vi "Puma_Ground_Control_Station_V2.1.vi"(0 "?":refnum<visa-resource-name>="COM3", 1 "?":u32=9600, 9 "XON":u8=17 format="%.0x", 14 "XOFF":u8=19 format="%.0x", 15 "?":u32=10000, 21 "?":bool=TRUE, 24 "?":u8=10 format="%.0x", 25 "bsize":u32=4096) -> ()   [LabVIEW 2015]
doc: "The Advanced Serial Read and Write example performs a Serial Port Read, a Serial Port Write, or a combination of these actions while setting some advanced serial features like buffer size, termination characters, and XON/XOFF flow control. The user selects the actions (read or write) on the front panel. If both are selected, the VI will write the data first, read the data and then close the VISA session that is opened to the port. \n\nThe parameters set for the serial port must match the parameters of the connected instrument or device. In this example, the bytes to read parameter specifies the number of bytes that the serial port reads. If there were more bytes at the port than the number specified in bytes to read, those bytes would not be read. Also, if you specify to read more bytes than the number of bytes actually read, you might receive a timeout error message.\n\nINSTRUCTIONS:\n1) Select the serial resource and configuration parameters (baud rate, data bits, parity, stop bits, flow control).\n2) Termination character can be enabled and set. Also, set the required input buffer size prior to running the example.\n3) Select the operations to be performed. \n4) Connect the serial port to your device. If no device is available, perform a loopback test by doing one of the following. Short pins 2 and 3 on a RS-232 cable or short pin 4 to pin 8 and pin 5 to pin 9 on a RS-485/422 cable. \n5) Run the VI to see the data read. (The \"read string\" will match the \"string to write\" if a loopback test was performed.)\n\nThis example exposes several advanced features that you may need for your application. Not all applications need all the features shown in this example. The input buffer size is likely an important setting that you want to control in your application. This example expands upon the flow control option for XON and XOFF, allowing the user to choose those control characters. The timeout parameter has been brought to the front panel so a user can specify the time period the VISA Read will wait for the number of bytes to read before timing out. Also, the user has several controls for the termination character, which is discussed later.\n\nNote that you can press the write and read buttons and change the bytes to read parameters on the fly, while the example is running. However, you must stop the example to change the other configuration parameters after the example has started running, and then run again.\n\nSet the I/O buffer size slightly higher the amount of data you expect to receive. This is very important for applications that don't use flow control, as you may lose characters if the receive buffer overflows.\n\nSetting the timeout period ensures that the operation returns with a timeout error if the operation cannot be performed in the specified time period. \n\nSome devices require a termination character in order to identify the end of command strings. Some devices send a termination character to signify the end of data to be read. \n\nThis example shows how you can end the Read operation once a termination character is detected in the buffer and/or append a termination character at the end of the Write data. To enable the Read to end on a termination character, use the VISA Configure Serial Port or use the VISA Properties Serial End Mode for Reads, Termination Character Enable, and Termination Character. To end the Write with a termination character, use the VISA Properties Serial End Mode for Writes, the Send End Enable, and Termination Character. In this example, the same termination character is used for both the Read and the Write. You can specify two different characters for your application, if desired.\n\nYour application may require specific characters for the XON/XOFF Flow Control. You can specify these characters with the VISA Properties Flow Control XOFF Character and Flow Control XON Character. Note that if the standard XON and XOFF characters are used, then decimal 17 and 19 are unavailable for data values. Remember that using flow control and setting an adequate buffer size allow you to prevent buffer overflows."
uses:
  <vilib>/Instr/_visa.llb/VISA Configure Serial Port (Instr).vi
panel:
  in  "Fan Shutdown":bool
  in  "DValve / AV6-T":bool
  in  "Flight Control Board":bool
  in  "Safety":bool
  in  "Test Run":bool
  in  "Reset Control":bool
  in  "Primary Safety 2":bool
  out "?":bool
  out "Motors":cluster{dbl, dbl, dbl, dbl}(graph)={1000.0, 1000.0, 1000.0, 1000.0}
  in  "Pressure Transducers":T1(tab)
  out "?":cluster{dbl, dbl, dbl, dbl, dbl}(graph)
  out "?":cluster{dbl, dbl}(graph)
  in  "Thermocouples":T2(tab)
  out "?":cluster{dbl, dbl, dbl, dbl}(graph)
  out "?":cluster{dbl, dbl}(graph)
  out "fo-u":bool
  out "av5-m":bool
  out "fc-u":bool
  out "PT1-U > 5000 PSI":bool
  out "Takeoff Started":bool
  out "Iterations":i32
  out "Reset Triggered":bool
  in  "PixHawk":bool
  in  "XON 2":u8=17 format="%.0x"
  in  "XOFF 2":u8=19 format="%.0x"
  in  "?":bool=TRUE
  in  "bsize 2":u32=4096
  in  "?":u8=10 format="%.0x"
  in  "?":bool=TRUE
  in  "?":u32=10000
  in  "?":refnum<visa-resource-name>="COM3"
  in  "?":u32=9600
  out "Max Values":T3={20.764332288, 0.0, 0.0, 0.0, 0.0, 0.0, 0.0, 201.058, 25.138999999999953, 0.0, 57.16000000000008, 0.0, 8.920000000000016, 15.403999999999996}
  in  "Data Filename":string
  out "Offset 7":dbl=-251.3
  out "Multiplier 7":dbl=1.264
  out "Offset 6":dbl=-250.2
  out "Offset 5":dbl=-250.3
  out "Offset 4":dbl=-1253.0
  out "Offset 3":dbl=-250.9
  out "Offset 2":dbl=-249.8
  out "Offset 1":dbl=-251.0
  out "Multiplier 6":dbl=1.264
  out "Multiplier 5":dbl=1.277
  out "Multiplier 4":dbl=6.36
  out "Multiplier 3":dbl=1.274
  out "Multiplier 2":dbl=1.267
  out "Multiplier 1":dbl=1.277
  in  "Begin Checklist":bool
  out "Manual Abort Tested":bool
  out "Flight Control On":bool
  out "Reset Triggered 2":bool
  out "Primary Safety Active":bool
  out "Craft Triggered Softkill Active":bool
  out "Hardkill Active":bool
  out "ms":dbl=163640.0
  out "vcc 6":bool
  out "gnd 6":bool=TRUE
  out "TC6":bool
  out "vcc 5":bool
  out "gnd 5":bool=TRUE
  out "TC5":bool
  out "vcc 4":bool
  out "gnd 4":bool=TRUE
  out "TC4":bool
  out "vcc 3":bool
  out "gnd 3":bool=TRUE
  out "TC3":bool
  out "vcc 2":bool
  out "gnd 2":bool=TRUE
  out "TC2":bool
  out "vcc":bool
  out "gnd":bool=TRUE
  out "TC1":bool
  out "Engine 4":dbl=1000.0
  out "Engine 3":dbl=1000.0
  out "Engine 2":dbl=1000.0
  out "Engine 1":dbl=1000.0
  out "soft kill ind":bool
  out "dump fuel ind":bool
  out "abort ind":bool
  out "run ind":bool
  out "av6-t ind":bool
  out "Control input":bool
  out "return":bool
  out "Control (on/off)":bool
  out "PT5-M":dbl=-6.084000000000003
  out "PT2-M":dbl=-10.039999999999992
  out "PT2-U":dbl=-250.3
  out "PT1-U":dbl=-38.24000000000001
  out "PT3-M":dbl=-141.336
  out "PT1-M":dbl=9.934999999999945
  out "PT4-M":dbl=181.90299999999996
  out "TCp-2":dbl=-2.0
  out "TCp-1":dbl=-2.0
  out "TCpw-4":dbl=-2.0
  out "TCpw-3":dbl=-2.0
  out "TCpw-2":dbl=-2.0
  out "TCpw-1":dbl=-2.0
  out "Output":string="h:;"
  in  "?":enum32{"Test"}(tab)
  in  "Primary Safety":bool=TRUE
  in  "Soft Kill":bool
  in  "Simulate":bool
  in  "Reset FC":bool
  in  "Full Power":bool
  in  "Secondary Safety":bool=TRUE
  in  "Takeoff":bool
  in  "Calibrate":bool
  in  "abort":bool
  out "?":dbl(graph)=20.40794784
  in  "Send":bool=TRUE
  in  "Recieve":bool=TRUE
  in  "bytes to read 2":u32=1000
  out "?":u32=107
  out "?":string[](array[string])=["339", "205", "86", "191", "0", "190", "194", "-2.00", "-2.00", "-2.00", "-2.00", "-2.00", "-2.00", "555", "1000", "1000", "1000", "1000", "163640"]
  out "?":string[](array[string])=["p:339,205,86,191,0,190,194", "t:-2.00,-2.00,-2.00,-2.00,-2.00,-2.00", "v:555", "m:1000,1000,1000,1000", "h:", "s:163640", ""]
  out "Voltage Sensor":dbl=20.40794784
  in  "dump fuel":bool
  in  "?":enum32{"Ignore"}(tab)
  out "?":bool=TRUE
  out "String":string
  in  "String 3":string
  in  "?":bool=TRUE
  in  "tank iso":bool
  in  "Av-6Tt":bool
  in  "FC-U Toggle":bool
  in  "FOU":bool
  out "?":dbl(slide) scale=0.2..200.0
  out "FO-U":bool
  out "FC-U":bool
  out "AV6-T":bool
  out "AV1-T":bool
  out "AV3-T":bool
  out "AV4-T":bool
  out "AV5-T":bool
  out "AV2-T":bool
  # "Data From Craft:"
  # "FO-U"
  # "FC-U"
  # "receive"
  # "send"
  # "AV6-M"
  # "AV5-M"
  # "green=open - check thermocouple attachments\nred=short gnd - contact Power or GNC\nblue=short vcc - contact Power or GNC"
  # "AV1-M"
  # "AV2-M"
  # "AV3-M"
  # "AV4-M"
  # "Voltage"
  # "TCp2-M"
  # "Tcw1-E"
  # "TCp1-M"
  # "TCw4-E"
  # "TCw3-E"
  # "TCw2-E"
  # "PT4-M"
  # "PT1-M"
  # "PT3-M"
  # "PT1-U"
  # "PT2-U"
  # "PT2-M"
  # "PT5-M"
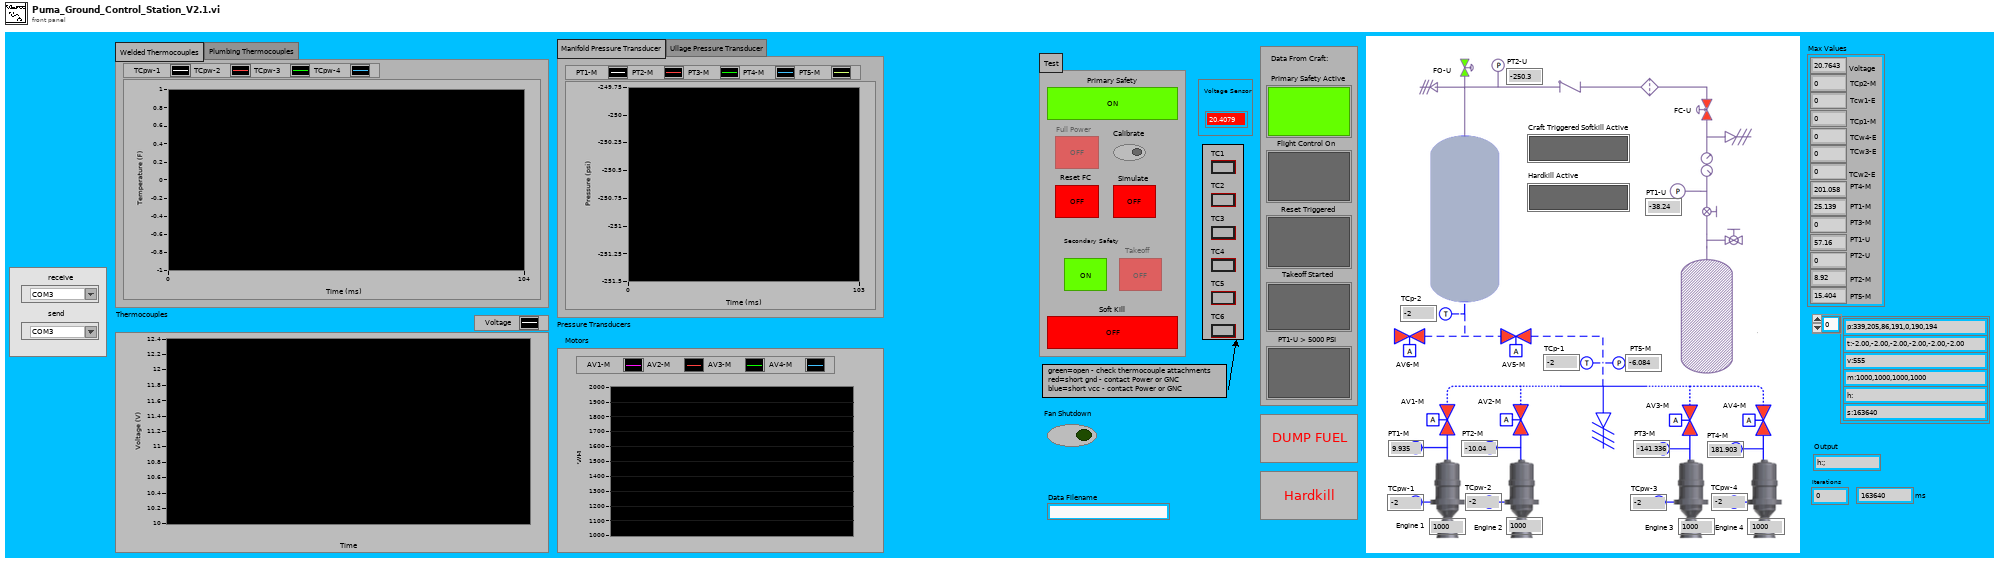
[diagram p1: front panel]
types:
  T1 = enum32{"Manifold Pressure Transducer", "Ullage Pressure Transducer"}
  T2 = enum32{"Welded Thermocouples", "Plumbing Thermocouples"}
  T3 = cluster{dbl, dbl, dbl, dbl, dbl, dbl, dbl, dbl, dbl, dbl, dbl, dbl, dbl, dbl}
  T4 = enum16{"open", "replace", "create", "open or create", "replace or create", "replace or create with confirmation"}
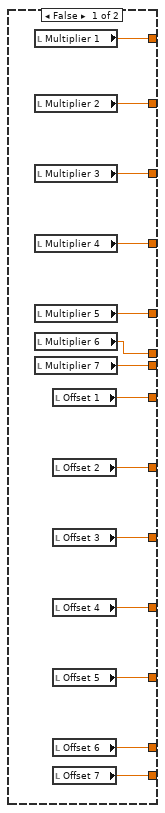
[diagram p3: hidden frame]
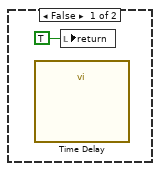
[diagram p13: hidden frame]
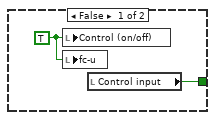
[diagram p16: hidden frame]
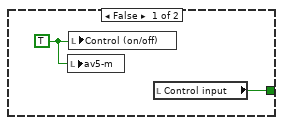
[diagram p18: hidden frame]
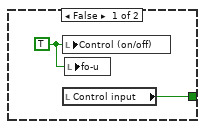
[diagram p20: hidden frame]
diagram:
  w2 = TRUE
  w1 = FALSE
  w51 = u16 16  # I/O Receive Buffer mask
  w75 = u16 16  # I/O Receive Buffer mask
  # "Comment"
  # "Set default values"
  n1 = while {
    stop <- FALSE stop-if-true
    n2 = case shown="True" "Calibrate" {
      tunnel: [w109 w123] -> w93
      tunnel: [w108 w122] -> w92
      tunnel: [w107 w121] -> w91
      tunnel: [w106 w120] -> w90
      tunnel: [w105 w119] -> w89
      tunnel: [w104 w118] -> w88
      tunnel: [w103 w117] -> w87
      tunnel: [w101 w116] -> w86
      tunnel: [w102 w115] -> w85
      tunnel: [w100 w114] -> w84
      tunnel: [w99 w113] -> w83
      tunnel: [w98 w112] -> w82
      tunnel: [w97 w111] -> w81
      tunnel: [w96 w110] -> w80
      frame False {
        n3 = local read "Multiplier 1"() -> (w109:dbl)
        n4 = local read "Multiplier 2"() -> (w108:dbl)
        n5 = local read "Multiplier 3"() -> (w107:dbl)
        n6 = local read "Multiplier 4"() -> (w106:dbl)
        n7 = local read "Multiplier 5"() -> (w105:dbl)
        n8 = local read "Multiplier 6"() -> (w104:dbl)
        n9 = local read "Multiplier 7"() -> (w103:dbl)
        n10 = local read "Offset 1"() -> (w101:dbl)
        n11 = local read "Offset 2"() -> (w102:dbl)
        n12 = local read "Offset 3"() -> (w100:dbl)
        n13 = local read "Offset 4"() -> (w99:dbl)
        n14 = local read "Offset 5"() -> (w98:dbl)
        n15 = local read "Offset 6"() -> (w97:dbl)
        n16 = local read "Offset 7"() -> (w96:dbl)
      }
      frame True {
        n17 = call "P configure.vi"() -> ("Multiplier 1"=w123:dbl, "Offset 1"=w116:dbl, "Multiplier 2"=w122:dbl, "Offset 2"=w115:dbl, "Multiplier 3"=w121:dbl, "Offset 6"=w111:dbl, "Offset 3"=w114:dbl, "Offset 7"=w110:dbl, "Multiplier 4"=w120:dbl, "Multiplier 7"=w117:dbl, "Multiplier 6"=w118:dbl, "Offset 5"=w112:dbl, "Multiplier 5"=w119:dbl, "Offset 4"=w113:dbl)  [unwired: 2 in]
      }
    }
    "Multiplier 1" <- w93
    "Multiplier 2" <- w92
    "Multiplier 3" <- w91
    "Multiplier 4" <- w90
    "Multiplier 5" <- w89
    "Offset 1" <- w86
    "Offset 2" <- w85
    "Offset 3" <- w84
    "Offset 4" <- w83
    "Offset 5" <- w82
    "Offset 6" <- w81
    "Multiplier 7" <- w87
    "Offset 7" <- w80
    "Multiplier 6" <- w88
  }
  n18 = while {
    stop <- FALSE stop-if-true
    n19 = local read "Control (on/off)"() -> (w126:bool)
    n20 = Wait Until Next ms Multiple(millisecond multiple=50) -> ()  [unwired: 1 out]
    n21 = case shown="True" w126 {
      frame False {
      }
      frame True {
        n22 = local read "dump fuel ind"() -> (w142:bool)
        n23 = local read "soft kill ind"() -> (w140:bool)
        n24 = local read "av6-t ind"() -> (w143:bool)
        n25 = local read "abort ind"() -> (w144:bool)
        n26 = local read "fc-u"() -> (w130:bool)
        n27 = local read "av5-m"() -> (w132:bool)
        n28 = local read "fo-u"() -> (w134:bool)
        n29 = local read "run ind"() -> (w141:bool)
        n30 = case shown="True" w140 {
          tunnel: [_ "Are you sure you want to Softkill?"] -> w135
          frame False {
          }
          frame True {
          }
        }
        n31 = case shown="True" w142 {
          tunnel: [_ "Are you sure you want to Dump Fuel?"] -> w137
          frame False {
          }
          frame True {
          }
        }
        n32 = case shown="True" w143 {
          tunnel: [_ "Are you sure you want to Open AV6-M?"] -> w138
          frame False {
          }
          frame True {
          }
        }
        n33 = case shown="True" w144 {
          tunnel: [_ "Are you sure you want to Abort?"] -> w139
          frame False {
          }
          frame True {
          }
        }
        n34 = case shown="True" w134 {
          tunnel: [_ "Are you sure you want to open FO-U?"] -> w133
          frame False {
          }
          frame True {
          }
        }
        n35 = case shown="True" w130 {
          tunnel: [_ "Are you sure you want to open FC-U?"] -> w129
          frame False {
          }
          frame True {
          }
        }
        n36 = case shown="True" w132 {
          tunnel: [_ "Are you sure you want to open AV5-M?"] -> w131
          frame False {
          }
          frame True {
          }
        }
        n37 = case shown="True" w141 {
          tunnel: [_ "Are you sure you want to Run?"] -> w136
          frame False {
          }
          frame True {
          }
        }
        n38 = Concatenate Strings(w135, w136, w137, w138, w139, w133, w131, w129) -> (w128:string)
        n39 = call "DialogBoxSubVI.vi"("Prompt"=w128) -> ("Boolean"=w127:bool)  [unwired: 9 in]
        n40 = case shown="True" w127 {
          frame False {
            n41 = call "Time Delay"() -> ()  [unwired: 11 in, 1 out]
            n42 = local write "return"(TRUE) -> ()
          }
          frame True {
            n43 = call "Time Delay2"() -> ()  [unwired: 11 in, 1 out]
            n44 = local write "return"(TRUE) -> ()
          }
        }
        n45 = local write "Control input"(w127) -> ()
      }
    }
  }
  n46 = call-poly "VISA Configure Serial Port"("VISA resource name"="?", "timeout (10sec)"="?", "termination char\n(0xA = '\\n' = LF)"="?", "Enable Termination\nChar (T)"="?", "baud rate (9600)"="?") -> ("VISA resource name out"=w64:refnum<visa-resource-name>, "error out"=w67:errorcluster)  [unwired: 5 in, 4 out]
  n47 = call-poly "VISA Configure Serial Port"("VISA resource name"="?", "timeout (10sec)"="?", "termination char\n(0xA = '\\n' = LF)"="?", "Enable Termination\nChar (T)"="?", "baud rate (9600)"="?") -> ("VISA resource name out"=w40:refnum<visa-resource-name>, "error out"=w43:errorcluster)  [unwired: 5 in, 4 out]
  n48 = case shown="True" "?" {
    selector: "?" -> [_ w157]
    tunnel: w64 -> [w155 w163]
    tunnel: w67 -> [w156 w162]
    tunnel: [w155 w161] -> w65
    tunnel: [w156 w160] -> w66
    tunnel: "?" -> [_ w158]
    frame False {
    }
    frame True {
      w159 = u16 2 items=["None", "LastBit", "TermChar", "Break"] ("Serial Settings:Serial End Mode for Writes")
      n49 = property class="Instr"(reference=w163, error in=w162, "Serial Settings:End Mode for Writes"=w159, "Message Based Settings:Send End Enable"=w157, "Message Based Settings:Termination Character"=w158) -> (reference out=w161:refnum<visa-resource-name>, error out=w160:errorcluster)
    }
  }
  n50 = case shown="True" "?" {
    selector: "?" -> [_ w166]
    tunnel: w40 -> [w164 w172]
    tunnel: w43 -> [w165 w171]
    tunnel: [w164 w170] -> w41
    tunnel: [w165 w169] -> w42
    tunnel: "?" -> [_ w167]
    frame False {
    }
    frame True {
      w168 = u16 2 items=["None", "LastBit", "TermChar", "Break"] ("Serial Settings:Serial End Mode for Writes")
      n51 = property class="Instr"(reference=w172, error in=w171, "Serial Settings:End Mode for Writes"=w168, "Message Based Settings:Send End Enable"=w166, "Message Based Settings:Termination Character"=w167) -> (reference out=w170:refnum<visa-resource-name>, error out=w169:errorcluster)
    }
  }
  n52 = property on="Secondary Safety" class="Bool (strict)"("Value"=w2) -> ()  [unwired: 2 in, 2 out]
  n53 = property on="Primary Safety" class="Bool (strict)"("Value"=w2) -> ()  [unwired: 2 in, 2 out]
  n54 = property on="Reset FC" class="Bool (strict)"("Value"=w1) -> ()  [unwired: 2 in, 2 out]
  n55 = property on="Simulate" class="Bool (strict)"("Value"=w1) -> ()  [unwired: 2 in, 2 out]
  n56 = property on="Craft Triggered Softkill Active" class="Bool (strict)"("Value"=w1) -> ()  [unwired: 2 in, 2 out]
  n57 = property on="Hardkill Active" class="Bool (strict)"("Value"=w1) -> ()  [unwired: 2 in, 2 out]
  n58 = property on="Takeoff Started" class="Bool (strict)"("Value"=w1) -> ()  [unwired: 2 in, 2 out]
  n59 = property on="FOU" class="Bool (strict)"("Value"=w1) -> ()  [unwired: 2 in, 2 out]
  n60 = property on="Soft Kill" class="Bool (strict)"("Value"=w1) -> ()  [unwired: 2 in, 2 out]
  n61 = property on="dump fuel" class="Bool (strict)"("Value"=w1) -> ()  [unwired: 2 in, 2 out]
  n62 = property on="abort" class="Bool (strict)"("Value"=w1) -> ()  [unwired: 2 in, 2 out]
  n63 = property on="Manual Abort Tested" class="Bool (strict)"("Value"=w1) -> ()  [unwired: 2 in, 2 out]
  n64 = Build Path(base path=path "C:/Users/Lunar Lion/Desktop/Puma_Test_Data" ("file path (use dialog)"), name or relative path="Data Filename") -> (appended path=w59:path)
  n65 = Build Array("PT4-M_a", "PT1-M_a", "PT3-M_a", "PT1-U_a", "PT2-U_a", "PT2-M_a", "PT5-M_a", "PT4-M", "PT1-M", "PT3-M", "PT1-U", "PT2-U", "PT2-M", "PT5-M", "TCp2-M", "TCw1-E", "TCp1-M", "TCw4-E", "TCw3-E", "TCw2-E", "Voltage", "Motor1", "Motor2", "Motor3", "Motor4", "Statestring") -> (w12:string[])
  n66 = VISA Set I/O Buffer Size(VISA resource name=w65, mask (16)=w75, size (4096)="bsize", error in (no error)=w66) -> (VISA resource name out=w71:refnum<visa-resource-name>, error out=w70:errorcluster)
  n67 = VISA Set I/O Buffer Size(VISA resource name=w41, mask (16)=w51, size (4096)="bsize 2", error in (no error)=w42) -> (VISA resource name out=w47:refnum<visa-resource-name>, error out=w46:errorcluster)
  n68 = Open/Create/Replace File(file path (use dialog)=w59, operation (0:open)=T4."replace or create with confirmation") -> (refnum out=w9:refnum<file>)  [unwired: 4 in, 2 out]
  n69 = Array To Spreadsheet String(array=w12, 3:"%s" ("format string")) -> (spreadsheet string=w10:string)  [unwired: 1 in]
  n70 = property class="Instr"(reference=w71, error in=w70, "Serial Settings:Flow Control XON Character"="XON", "Serial Settings:Flow Control XOFF Character"="XOFF") -> (reference out=w63:refnum<visa-resource-name>, error out=w62:errorcluster)
  n71 = property class="Instr"(reference=w47, error in=w46, "Serial Settings:Flow Control XON Character"="XON 2", "Serial Settings:Flow Control XOFF Character"="XOFF 2") -> (reference out=w39:refnum<visa-resource-name>)  [unwired: 1 out]
  n72 = Write to Text File(file (use dialog)=w9, text=w10) -> (refnum out=w8:refnum<file>)  [unwired: 2 in, 2 out]
  n73 = while {
    tunnel: w63 -> [w304]
    tunnel: w62 -> [w373]
    tunnel: [w283] -> w7
    tunnel: [w282] -> w61
    shift-right: [w473] -> _
    shift-left: _ -> [w472]
    shift-right: [w184] -> _
    shift-left: _ -> [w434]
    shift-right: [w442] -> _
    shift-left: _ -> [w443]
    shift-right: [w433] -> _
    shift-left: _ -> [w457]
    shift-right: [w187] -> _
    shift-left: _ -> [w455]
    shift-right: [w435] -> _
    shift-left: _ -> [w438]
    shift-right: ["Begin Checklist"] -> _
    shift-left: _ -> [w354]
    tunnel: w8 -> [w326]
    tunnel: [w323] -> w58
    shift-right: [w307] -> _
    shift-left: T3 {0.0, 0.0, 0.0, 0.0, 0.0, 0.0, 0.0, 0.0, 0.0, 0.0, 0.0, 0.0, 0.0, 0.0} -> [w306]
    tunnel: w39 -> [_]
    shift-right: [w182] -> _
    shift-left: _ -> [w186]
    shift-right: [w179] -> _
    shift-left: _ -> [w180]
    shift-right: [w176] -> _
    shift-left: _ -> [w177]
    i -> [w292]
    stop <- FALSE stop-if-true
    w208 = u32 13816530
    w212 = 120.0
    w218 = 1200.0
    w209 = u32 16776704
    w225 = 800.0
    # "The purpose of this indicator is not entirely clear"
    # "Hidden test run button."
    # "Hidden secondary safety."
    # "Hidden reset control button."
    # "Hidden flight control board button."
    # "Un-named indicator, hidden."
    # "Hidden dump valve indicator/button?"
    # "Hidden primary safety"
    # "Tabs for the main command buttons."
    # "Ignore tab with the two strings and indicator light."
    # "Above nominal thresholds:\n   All PTs except PT1-U: 800\n   TCpw-1 to 4: 1200\n   TCp-1 and 2: 120"
    # "The second String \nParsing Indicator"
    # "String Parsing Indicator control"
    # "ENSURE THE PTs ARE HOOKED UP PROPERLY"
    # "Here, if PT1-U indicates a pressure greater than 5000 psi,\nthe indicator represented in the case structure is turned green. Otherwise, it is turned red."
    # "FO-U Case"
    # "AV6 -T Case"
    # "AV5-T Case"
    # "AV5-T Toggle"
    n74 = case shown="True" FALSE {
      frame False {
      }
      frame True {
        w589 = FALSE
        n75 = local write "FOU"(TRUE) -> ()
        n76 = local write "AV1-T"(w589) -> ()
        n77 = local write "AV2-T"(w589) -> ()
        n78 = local write "AV3-T"(w589) -> ()
        n79 = local write "AV4-T"(w589) -> ()
        n80 = local write "FC-U Toggle"(w589) -> ()
        n81 = local write "tank iso"(w589) -> ()
      }
    }
    n82 = property on="abort" class="Bool (strict)"() -> ("Value"=w260:bool)  [unwired: 2 in, 2 out]
    n83 = property on="Voltage Sensor" class="DigNum (strict)"("NumText.TextColor"=u32 16448250) -> ()  [unwired: 2 in, 2 out]
    n84 = local read "Voltage Sensor"() -> (w264:dbl)
    n85 = case shown="False" w260 {
      frame False {
        n86 = property on="Soft Kill" class="Bool (strict)"() -> ("Value"=w573:bool)  [unwired: 2 in, 2 out]
        n87 = case shown="True" w573 {
          frame False {
            n88 = property on="dump fuel" class="Bool (strict)"("DisabledEnum"=0) -> ()  [unwired: 2 in, 2 out]
          }
          frame True {
            n89 = property on="dump fuel" class="Bool (strict)"("DisabledEnum"=2) -> ()  [unwired: 2 in, 2 out]
          }
        }
      }
      frame True {
        n90 = property on="dump fuel" class="Bool (strict)"("DisabledEnum"=2) -> ()  [unwired: 2 in, 2 out]
      }
    }
    n91 = Greater Than 0?(x=w264) -> (x > 0?=w271:bool)
    n92 = Less?(x=w264, y=14.0) -> (x < y?=w277:bool)
    n93 = Less?(x=w264, y=13.0) -> (x < y?=w272:bool)
    n94 = Greater?(x=w264, y=13.0) -> (0:w276:bool)
    n95 = Greater?(x=w264, y=14.0) -> (0:w268:bool)
    n96 = Less?(x=w264, y=15.5) -> (x < y?=w269:bool)
    n97 = Greater?(x=w264, y=15.5) -> (0:w263:bool)
    n98 = And(x=w268, y=w269) -> (x .and. y?=w267:bool)
    n99 = And(x=w271, y=w272) -> (x .and. y?=w273:bool)
    n100 = And(x=w276, y=w277) -> (x .and. y?=w278:bool)
    n101 = case shown="True" w273 {
      frame False {
      }
      frame True {
        n102 = property on="Voltage Sensor" class="DigNum (strict)"("NumText.BGColor"=u32 16714752) -> ()  [unwired: 2 in, 2 out]
      }
    }
    n103 = case shown="True" w278 {
      frame False {
      }
      frame True {
        n104 = property on="Voltage Sensor" class="DigNum (strict)"("NumText.BGColor"=u32 16757522) -> ()  [unwired: 2 in, 2 out]
        n105 = property on="Voltage Sensor" class="DigNum (strict)"("NumText.TextColor"=u32 16777222) -> ()  [unwired: 2 in, 2 out]
      }
    }
    n106 = case shown="True" w267 {
      frame False {
      }
      frame True {
        n107 = property on="Voltage Sensor" class="DigNum (strict)"("NumText.BGColor"=u32 6618880) -> ()  [unwired: 2 in, 2 out]
        n108 = property on="Voltage Sensor" class="DigNum (strict)"("NumText.TextColor"=u32 16777222) -> ()  [unwired: 2 in, 2 out]
      }
    }
    n109 = case shown="True" w263 {
      frame False {
      }
      frame True {
        n110 = property on="Voltage Sensor" class="DigNum (strict)"("NumText.BGColor"=u32 15876863) -> ()  [unwired: 2 in, 2 out]
      }
    }
    n111 = Exclusive Or(1:w457, 2:"abort") -> (0:w459:bool)
    n112 = case shown="True" w459 {
      tunnel: [w653 w655] -> w433
      tunnel: w457 -> [w653 w654]
      frame False {
      }
      frame True {
        n113 = case shown="False" w654 {
          tunnel: [w656 FALSE ("T button?")] -> w655
          frame False {
            w657 = TRUE
            n114 = local write "abort ind"(w657) -> ()
            n115 = local write "Control (on/off)"(w657) -> ()
            n116 = local read "Control input"() -> (w656:bool)
          }
          frame True {
          }
        }
      }
    }
    n117 = Exclusive Or(1:w438, 2:"Soft Kill") -> (0:w436:bool)
    n118 = Exclusive Or(1:w455, 2:"dump fuel") -> (0:w456:bool)
    n119 = case shown="True" w436 {
      tunnel: [w643 w645] -> w435
      tunnel: w438 -> [w643 w644]
      frame False {
      }
      frame True {
        n120 = case shown="False" w644 {
          tunnel: [w646 _] -> w645
          frame False {
            w647 = TRUE
            n121 = local write "soft kill ind"(w647) -> ()
            n122 = local write "Control (on/off)"(w647) -> ()
            n123 = local read "Control input"() -> (w646:bool)
          }
          frame True {
          }
        }
      }
    }
    n124 = case shown="True" w456 {
      tunnel: [w648 w650] -> w187
      tunnel: w455 -> [w648 w649]
      frame False {
      }
      frame True {
        n125 = case shown="False" w649 {
          tunnel: [w652 _] -> w650
          frame False {
            w651 = TRUE
            n126 = local write "Control (on/off)"(w651) -> ()
            n127 = local write "dump fuel ind"(w651) -> ()
            n128 = local read "Control input"() -> (w652:bool)
          }
          frame True {
          }
        }
      }
    }
    n129 = Not(x="Secondary Safety") -> (.not. x?=w293:bool)
    n130 = property on="TCpw-1" class="DigNum (strict)"() -> ("Value"=w222:dbl)  [unwired: 2 in, 2 out]
    n131 = property on="TCpw-2" class="DigNum (strict)"() -> ("Value"=w217:dbl)  [unwired: 2 in, 2 out]
    n132 = property on="TCpw-3" class="DigNum (strict)"() -> ("Value"=w216:dbl)  [unwired: 2 in, 2 out]
    n133 = property on="TCpw-4" class="DigNum (strict)"() -> ("Value"=w215:dbl)  [unwired: 2 in, 2 out]
    n134 = property on="TCp-2" class="DigNum (strict)"() -> ("Value"=w210:dbl)  [unwired: 2 in, 2 out]
    n135 = property on="TCp-1" class="DigNum (strict)"() -> ("Value"=w211:dbl)  [unwired: 2 in, 2 out]
    n136 = property on="PT2-M" class="DigNum (strict)"() -> ("Value"=w235:dbl)  [unwired: 2 in, 2 out]
    n137 = property on="PT1-M" class="DigNum (strict)"() -> ("Value"=w236:dbl)  [unwired: 2 in, 2 out]
    n138 = property on="PT3-M" class="DigNum (strict)"() -> ("Value"=w234:dbl)  [unwired: 2 in, 2 out]
    n139 = property on="PT4-M" class="DigNum (strict)"() -> ("Value"=w233:dbl)  [unwired: 2 in, 2 out]
    n140 = property on="PT5-M" class="DigNum (strict)"() -> ("Value"=w227:dbl)  [unwired: 2 in, 2 out]
    n141 = property on="PT2-U" class="DigNum (strict)"() -> ("Value"=w226:dbl)  [unwired: 2 in, 2 out]
    n142 = And(x="Safety", y="Test Run") -> (x .and. y?=w488:bool)
    n143 = And(x=w293, y="Takeoff") -> (x .and. y?=w487:bool)
    n144 = Not(x="Secondary Safety") -> (.not. x?=w295:bool)
    n145 = Greater Or Equal?(x=w210, y=w212) -> (x >= y?=w213:bool)
    n146 = Greater Or Equal?(x=w211, y=w212) -> (x >= y?=w214:bool)
    n147 = Greater Or Equal?(x=w222, y=w218) -> (x >= y?=w223:bool)
    n148 = Greater Or Equal?(x=w217, y=w218) -> (x >= y?=w221:bool)
    n149 = Greater Or Equal?(x=w216, y=w218) -> (x >= y?=w220:bool)
    n150 = Greater Or Equal?(x=w215, y=w218) -> (x >= y?=w219:bool)
    n151 = Greater Or Equal?(x=w235, y=w225) -> (x >= y?=w231:bool)
    n152 = Greater Or Equal?(x=w236, y=w225) -> (x >= y?=w232:bool)
    n153 = Greater Or Equal?(x=w234, y=w225) -> (x >= y?=w230:bool)
    n154 = Greater Or Equal?(x=w233, y=w225) -> (x >= y?=w229:bool)
    n155 = Greater Or Equal?(x=w227, y=w225) -> (x >= y?=w228:bool)
    n156 = Greater Or Equal?(x=w226, y=w225) -> (x >= y?=w224:bool)
    n157 = case shown="True" "Recieve" {
      tunnel: w373 -> [w707 w712]
      tunnel: w304 -> [w708 w711]
      tunnel: [w707 w714] -> w282
      tunnel: [w708 w713] -> w283
      tunnel: [_ w710] -> _
      tunnel: [_ w709] -> w325
      frame False {
      }
      frame True {
        n158 = case "Read bytes from port." shown="No Error" w712 {
          selector: w712 -> [w717 w723]
          tunnel: [w720 w723] -> w714
          tunnel: [w721 w722] -> w713
          tunnel: w711 -> [w718 w722]
          tunnel: [w715 _] -> w710
          tunnel: [w715 _] -> w709
          frame No Error {
            n159 = VISA Read(VISA resource name=w718, byte count="bytes to read 2", error in (no error)=w717) -> (VISA resource name out=w721:refnum<visa-resource-name>, read buffer=w715:string, return count=→"?":u32, error out=w720:errorcluster)
          }
          frame Error {
          }
        }
      }
    }
    n160 = case shown="False" w295 {
      tunnel: [2 0] -> w294
      frame False {
      }
      frame True {
      }
    }
    n161 = Or(x=w487, y=w488) -> (x .or. y?=w462:bool)
    n162 = case shown="True" w213 {
      tunnel: w209 -> [_ w550]
      tunnel: w208 -> [w549 _]
      frame False {
        n163 = property on="TCp-2" class="DigNum (strict)"("NumText.BGColor"=w549) -> ()  [unwired: 2 in, 2 out]
      }
      frame True {
        n164 = property on="TCp-2" class="DigNum (strict)"("NumText.BGColor"=w550) -> ()  [unwired: 2 in, 2 out]
      }
    }
    n165 = case shown="True" w214 {
      tunnel: w209 -> [_ w552]
      tunnel: w208 -> [w551 _]
      frame False {
        n166 = property on="TCp-1" class="DigNum (strict)"("NumText.BGColor"=w551) -> ()  [unwired: 2 in, 2 out]
      }
      frame True {
        n167 = property on="TCp-1" class="DigNum (strict)"("NumText.BGColor"=w552) -> ()  [unwired: 2 in, 2 out]
      }
    }
    n168 = case shown="True" w223 {
      tunnel: w209 -> [_ w560]
      tunnel: w208 -> [w559 _]
      frame False {
        n169 = property on="TCpw-1" class="DigNum (strict)"("NumText.BGColor"=w559) -> ()  [unwired: 2 in, 2 out]
      }
      frame True {
        n170 = property on="TCpw-1" class="DigNum (strict)"("NumText.BGColor"=w560) -> ()  [unwired: 2 in, 2 out]
      }
    }
    n171 = case shown="True" w221 {
      tunnel: w209 -> [_ w558]
      tunnel: w208 -> [w557 _]
      frame False {
        n172 = property on="TCpw-2" class="DigNum (strict)"("NumText.BGColor"=w557) -> ()  [unwired: 2 in, 2 out]
      }
      frame True {
        n173 = property on="TCpw-2" class="DigNum (strict)"("NumText.BGColor"=w558) -> ()  [unwired: 2 in, 2 out]
      }
    }
    n174 = case shown="True" w220 {
      tunnel: w209 -> [_ w556]
      tunnel: w208 -> [w555 _]
      frame False {
        n175 = property on="TCpw-3" class="DigNum (strict)"("NumText.BGColor"=w555) -> ()  [unwired: 2 in, 2 out]
      }
      frame True {
        n176 = property on="TCpw-3" class="DigNum (strict)"("NumText.BGColor"=w556) -> ()  [unwired: 2 in, 2 out]
      }
    }
    n177 = case shown="True" w219 {
      tunnel: w209 -> [_ w554]
      tunnel: w208 -> [w553 _]
      frame False {
        n178 = property on="TCpw-4" class="DigNum (strict)"("NumText.BGColor"=w553) -> ()  [unwired: 2 in, 2 out]
      }
      frame True {
        n179 = property on="TCpw-4" class="DigNum (strict)"("NumText.BGColor"=w554) -> ()  [unwired: 2 in, 2 out]
      }
    }
    n180 = case shown="True" w231 {
      tunnel: w209 -> [_ w570]
      tunnel: w208 -> [w569 _]
      frame False {
        n181 = property on="PT2-M" class="DigNum (strict)"("NumText.BGColor"=w569) -> ()  [unwired: 2 in, 2 out]
      }
      frame True {
        n182 = property on="PT2-M" class="DigNum (strict)"("NumText.BGColor"=w570) -> ()  [unwired: 2 in, 2 out]
      }
    }
    n183 = case shown="True" w232 {
      tunnel: w209 -> [_ w572]
      tunnel: w208 -> [w571 _]
      frame False {
        n184 = property on="PT1-M" class="DigNum (strict)"("NumText.BGColor"=w571) -> ()  [unwired: 2 in, 2 out]
      }
      frame True {
        n185 = property on="PT1-M" class="DigNum (strict)"("NumText.BGColor"=w572) -> ()  [unwired: 2 in, 2 out]
      }
    }
    n186 = case shown="True" w230 {
      tunnel: w209 -> [_ w568]
      tunnel: w208 -> [w567 _]
      frame False {
        n187 = property on="PT3-M" class="DigNum (strict)"("NumText.BGColor"=w567) -> ()  [unwired: 2 in, 2 out]
      }
      frame True {
        n188 = property on="PT3-M" class="DigNum (strict)"("NumText.BGColor"=w568) -> ()  [unwired: 2 in, 2 out]
      }
    }
    n189 = case shown="True" w229 {
      tunnel: w209 -> [_ w566]
      tunnel: w208 -> [w565 _]
      frame False {
        n190 = property on="PT4-M" class="DigNum (strict)"("NumText.BGColor"=w565) -> ()  [unwired: 2 in, 2 out]
      }
      frame True {
        n191 = property on="PT4-M" class="DigNum (strict)"("NumText.BGColor"=w566) -> ()  [unwired: 2 in, 2 out]
      }
    }
    n192 = case shown="True" w228 {
      tunnel: w209 -> [_ w564]
      tunnel: w208 -> [w563 _]
      frame False {
        n193 = property on="PT5-M" class="DigNum (strict)"("NumText.BGColor"=w563) -> ()  [unwired: 2 in, 2 out]
      }
      frame True {
        n194 = property on="PT5-M" class="DigNum (strict)"("NumText.BGColor"=w564) -> ()  [unwired: 2 in, 2 out]
      }
    }
    n195 = case shown="True" w224 {
      tunnel: w209 -> [_ w562]
      tunnel: w208 -> [w561 _]
      frame False {
        n196 = property on="PT2-U" class="DigNum (strict)"("NumText.BGColor"=w561) -> ()  [unwired: 2 in, 2 out]
      }
      frame True {
        n197 = property on="PT2-U" class="DigNum (strict)"("NumText.BGColor"=w562) -> ()  [unwired: 2 in, 2 out]
      }
    }
    n198 = Exclusive Or(1:w434, 2:w462) -> (0:w461:bool)
    n199 = case shown="True" w461 {
      tunnel: [w659 w661] -> w184
      tunnel: w434 -> [w659 w660]
      frame False {
      }
      frame True {
        n200 = case shown="True" w660 {
          tunnel: [w663 _] -> w661
          frame False {
            w662 = TRUE
            n201 = local write "run ind"(w662) -> ()
            n202 = local write "Control (on/off)"(w662) -> ()
            n203 = local read "Control input"() -> (w663:bool)
          }
          frame True {
            w664 = FALSE
            n204 = local write "Test Run"(w664) -> ()
            n205 = local write "Control (on/off)"(w664) -> ()
            n206 = local write "Takeoff"(w664) -> ()
          }
        }
      }
    }
    "AV1-T" <- w184
    "AV4-T" <- w184
    "AV2-T" <- w184
    "AV3-T" <- w184
    n207 = case shown="True" "FC-U Toggle" {
      tunnel: [w531 w533] -> w176
      tunnel: w177 -> [w531 w532]
      frame False {
      }
      frame True {
        n208 = case shown="True" w532 {
          tunnel: [w534 _] -> w533
          frame False {
            w535 = TRUE
            n209 = local write "Control (on/off)"(w535) -> ()
            n210 = local write "fc-u"(w535) -> ()
            n211 = local read "Control input"() -> (w534:bool)
          }
          frame True {
            n212 = local write "FC-U Toggle"(FALSE) -> ()
          }
        }
      }
    }
    "FC-U" <- w176
    n213 = case shown="True" "tank iso" {
      tunnel: [w537 w539] -> w179
      tunnel: w180 -> [w537 w538]
      frame False {
      }
      frame True {
        n214 = case shown="True" w538 {
          tunnel: [w540 _] -> w539
          frame False {
            w541 = TRUE
            n215 = local write "av5-m"(w541) -> ()
            n216 = local write "Control (on/off)"(w541) -> ()
            n217 = local read "Control input"() -> (w540:bool)
          }
          frame True {
            n218 = local write "tank iso"(FALSE) -> ()
          }
        }
      }
    }
    "AV5-T" <- w179
    n219 = property on="Takeoff" class="Bool (strict)"("DisabledEnum"=w294) -> ()  [unwired: 2 in, 2 out]
    n220 = case shown="True" "FOU" {
      tunnel: [w543 w545] -> w182
      tunnel: w186 -> [w543 w544]
      frame False {
      }
      frame True {
        n221 = case shown="True" w544 {
          tunnel: [w546 _] -> w545
          frame False {
            w547 = TRUE
            n222 = local write "Control (on/off)"(w547) -> ()
            n223 = local read "Control input"() -> (w546:bool)
            n224 = local write "fo-u"(w547) -> ()
          }
          frame True {
            n225 = local write "FOU"(FALSE) -> ()
          }
        }
      }
    }
    "FO-U" <- w182
    n226 = Or(x=w433, y=w435) -> (x .or. y?=w460:bool)
    n227 = Or(x=w460, y=w187) -> (x .or. y?=w430:bool)
    n228 = Not(x=w430) -> (.not. x?=w262:bool)
    n229 = And(x=w262, y="Safety") -> (x .and. y?=w447:bool)
    n230 = And(x=w262, y="Test Run") -> (x .and. y?=w444:bool)
    n231 = And(x=w262, y="Secondary Safety") -> (x .and. y?=w446:bool)
    n232 = And(x=w262, y="Takeoff") -> (x .and. y?=w445:bool)
    n233 = local write "Safety"(w447) -> ()
    n234 = local write "Test Run"(w444) -> ()
    n235 = local write "Takeoff"(w445) -> ()
    n236 = Concatenate Strings(w325, "\n" ("string")) -> ()  [unwired: 1 out]
    n237 = Or(x=w447, y=w446) -> (x .or. y?=w450:bool)
    n238 = Or(x=w445, y=w444) -> (x .or. y?=w449:bool)
    n239 = Spreadsheet String To Array(delimiter (Tab)=";", format string="%d", spreadsheet string=w325, array type (2D Dbl)=string[] ["p:1234.1234.1234.1234,1234,1234", "t:1234,1234,1234"] ("Array of Strings 3")) -> (array=w526:string[])
    "?" <- w526
    n240 = Or(x=w450, y=w449) -> (x .or. y?=w448:bool)
    n241 = Or(x="Av-6Tt", y="DValve / AV6-T") -> (x .or. y?=w439:bool)
    n242 = Or(x="Reset Control", y="Reset FC") -> (x .or. y?=w474:bool)
    n243 = Or(x=w182, y=w184) -> (x .or. y?=w183:bool)
    n244 = local read "return"() -> (w453:bool)
    n245 = case shown="True" w439 {
      tunnel: [w637 w638] -> w442
      tunnel: w443 -> [w637 w639]
      frame False {
      }
      frame True {
        n246 = case shown="False" w639 {
          tunnel: [w641 _] -> w638
          frame False {
            w640 = TRUE
            n247 = local write "Control (on/off)"(w640) -> ()
            n248 = local write "av6-t ind"(w640) -> ()
            n249 = local read "Control input"() -> (w641:bool)
          }
          frame True {
            w642 = FALSE
            n250 = local write "Av-6Tt"(w642) -> ()
            n251 = local write "DValve / AV6-T"(w642) -> ()
          }
        }
      }
    }
    "AV6-T" <- w442
    "?" <- w442
    n252 = case shown="True" w184 {
      tunnel: [_ "o" ("write buffer")] -> w492
      tunnel: w472 -> [w677 w685]
      tunnel: [w678 w681] -> w473
      tunnel: w474 -> [w676 _]
      frame False {
        n253 = case shown="False" w676 {
          tunnel: [w679 200.0] -> w678
          tunnel: w677 -> [w679 _]
          frame False {
          }
          frame True {
          }
        }
      }
      frame True {
        # "Send 'o' Takeoff"
        n254 = Subtract(x=w685, y=0.0) -> (x-y=w682:dbl)
        n255 = Greater Than 0?(x=w682) -> (x > 0?=w683:bool)
        n256 = case shown="True" w683 {
          selector: w683 -> [_ w691]
          tunnel: w682 -> [_ w692]
          tunnel: [w687 w692] -> w681
          frame False {
            n257 = local read "Takeoff Started"() -> (w688:bool)
            n258 = case shown="False" w688 {
              tunnel: [200.0 0.0] -> w687
              frame False {
              }
              frame True {
              }
            }
          }
          frame True {
            "Takeoff Started" <- w691
          }
        }
      }
    }
    "?" <- w473
    n259 = Or(x=w183, y=w448) -> (x .or. y?=w451:bool)
    n260 = Array Size(array=w526) -> (size(s)=w527:i32)
    n261 = for {
      N: w527 -> [_]
      tunnel: w526 -> [w732]
      tunnel: [w724] -> w471 mode=concatenating
      i -> [w731]
      n262 = Index Array(array=w732, index=w731) -> (element=w727:string)
      n263 = String Subset(string=w727, offset (0)=2) -> (substring=w725:string)  [unwired: 1 in]
      n264 = Spreadsheet String To Array(delimiter (Tab)=",", format string="%d", spreadsheet string=w725, array type (2D Dbl)=string[] ["p:1234.1234.1234.1234,1234,1234", "t:1234,1234,1234"] ("Array of Strings 3")) -> (array=w724:string[])
    }
    n265 = Or(x=w453, y=w451) -> (x .or. y?=w454:bool)
    n266 = And(x=w453, y=w454) -> (x .and. y?=w452:bool)
    n267 = case shown="True" w452 {
      tunnel: w184 -> [_ w600]
      tunnel: w435 -> [_ w603]
      tunnel: w434 -> [_ w602]
      tunnel: [_ w601] -> _
      tunnel: w187 -> [_ w601]
      tunnel: w433 -> [_ w599]
      tunnel: w182 -> [_ w597]
      tunnel: w179 -> [_ w596]
      tunnel: w176 -> [_ w593]
      frame False {
      }
      frame True {
        n268 = local read "fc-u"() -> (w594:bool)
        n269 = case shown="True" w600 {
          frame False {
            w635 = FALSE
            n270 = local write "return"(w635) -> ()
            n271 = local write "Control (on/off)"(w635) -> ()
            n272 = local write "Control input"(w635) -> ()
          }
          frame True {
            w636 = FALSE
            n273 = local write "return"(w636) -> ()
            n274 = local write "Control (on/off)"(w636) -> ()
            n275 = local write "Control input"(w636) -> ()
          }
        }
        n276 = case shown="True" w594 {
          tunnel: w593 -> [_ w610]
          frame False {
          }
          frame True {
            n277 = local write "fc-u"(FALSE) -> ()
            n278 = case shown="False" w610 {
              frame False {
                n279 = local write "FC-U Toggle"(FALSE) -> ()
              }
              frame True {
                n280 = local write "FC-U Toggle"(FALSE) -> ()
              }
            }
          }
        }
        n281 = local read "soft kill ind"() -> (w608:bool)
        n282 = local read "abort ind"() -> (w605:bool)
        n283 = local read "av6-t ind"() -> (w604:bool)
        n284 = local read "run ind"() -> (w606:bool)
        n285 = local read "dump fuel ind"() -> (w607:bool)
        n286 = local read "fo-u"() -> (w598:bool)
        n287 = case shown="True" w605 {
          tunnel: w599 -> [_ w627]
          frame False {
          }
          frame True {
            n288 = local write "abort"(w627) -> ()
            n289 = local write "abort ind"(FALSE) -> ()
          }
        }
        n290 = case shown="True" w608 {
          tunnel: w600 -> [_ _]
          tunnel: w603 -> [_ w629]
          frame False {
          }
          frame True {
            n291 = local write "Soft Kill"(w629) -> ()
            n292 = local write "soft kill ind"(FALSE) -> ()
          }
        }
        n293 = case shown="True" w606 {
          tunnel: w600 -> [_ w634]
          frame False {
          }
          frame True {
            n294 = local write "Takeoff"(w634) -> ()
            n295 = local write "Test Run"(w634) -> ()
            n296 = local write "run ind"(FALSE) -> ()
          }
        }
        n297 = case shown="True" w604 {
          tunnel: w602 -> [_ w622]
          frame False {
          }
          frame True {
            n298 = case shown="True" w622 {
              frame False {
                n299 = local write "Av-6Tt"(FALSE) -> ()
                n300 = local write "DValve / AV6-T"(FALSE) -> ()
              }
              frame True {
                n301 = local write "Av-6Tt"(FALSE) -> ()
                n302 = local write "DValve / AV6-T"(FALSE) -> ()
              }
            }
            n303 = local write "av6-t ind"(FALSE) -> ()
          }
        }
        n304 = case shown="True" w607 {
          tunnel: w601 -> [_ w631]
          frame False {
          }
          frame True {
            n305 = local write "dump fuel"(w631) -> ()
            n306 = local write "dump fuel ind"(FALSE) -> ()
          }
        }
        n307 = case shown="True" w598 {
          tunnel: w597 -> [_ w617]
          frame False {
          }
          frame True {
            n308 = case shown="True" w617 {
              frame False {
                n309 = local write "FOU"(FALSE) -> ()
              }
              frame True {
                n310 = local write "FOU"(FALSE) -> ()
              }
            }
            n311 = local write "fo-u"(FALSE) -> ()
          }
        }
        n312 = local read "av5-m"() -> (w595:bool)
        n313 = case shown="True" w595 {
          tunnel: w596 -> [_ w613]
          frame False {
          }
          frame True {
            n314 = case shown="False" w613 {
              frame False {
                n315 = local write "tank iso"(FALSE) -> ()
              }
              frame True {
                n316 = local write "tank iso"(FALSE) -> ()
              }
            }
            n317 = local write "av5-m"(FALSE) -> ()
          }
        }
      }
    }
    n318 = Not(x="Primary Safety") -> ()  [unwired: 1 out]
    n319 = case shown="False" "Primary Safety" {
      tunnel: [0 2] -> w291
      tunnel: [w583 FALSE] -> w288
      frame False {
        n320 = property on="Full Power" class="Bool (strict)"() -> ("Value"=w583:bool)  [unwired: 2 in, 2 out]
      }
      frame True {
      }
    }
    n321 = Not(x="Primary Safety") -> (.not. x?=w297:bool)
    n322 = case shown="True" "PixHawk" {
      tunnel: [_ "y" ("write buffer")] -> w494
      frame False {
      }
      frame True {
        # "Send 'y' Turn on Pixhawk"
      }
    }
    n323 = case shown="True" w297 {
      tunnel: [_ "s" ("write buffer")] -> w498
      frame False {
      }
      frame True {
        # "Send 's' to disengage safety"
      }
    }
    n324 = case shown="True" w474 {
      tunnel: [_ "r" ("write buffer")] -> w496
      frame False {
      }
      frame True {
        # "Send 'r' Reset Flight Computer"
      }
    }
    n325 = case shown="True" "Simulate" {
      tunnel: [_ "p" ("write buffer")] -> w493
      frame False {
      }
      frame True {
        # "Send 'p' begin flight profile sim"
      }
    }
    n326 = case shown="False" "Simulate" {
      tunnel: w471 -> [w665 w666]
      tunnel: [w665 w666] -> w376
      tunnel: [_ w666] -> w470
      frame False {
      }
      frame True {
      }
    }
    "?" <- w376
    n327 = Or(x="Flight Control Board", y="Full Power") -> (x .or. y?=w484:bool)
    n328 = case shown="True" w182 {
      tunnel: [_ "d"] -> w483
      frame False {
      }
      frame True {
      }
    }
    n329 = case shown="True" w484 {
      tunnel: [_ "z" ("write buffer")] -> w497
      frame False {
      }
      frame True {
        # "Send 'z' Turn on Power"
      }
    }
    n330 = case shown="True" w187 {
      tunnel: [_ "b" ("write buffer")] -> w479
      frame False {
      }
      frame True {
        # "Send 'b' Dump FUEL"
      }
    }
    n331 = case shown="True" w442 {
      tunnel: [_ "v" ("write buffer")] -> w480
      frame False {
      }
      frame True {
        # "Send 'v' Dump Valve"
      }
    }
    n332 = property on="Full Power" class="Bool (strict)"("Value"=w288) -> ()  [unwired: 2 in, 2 out]
    n333 = property on="Full Power" class="Bool (strict)"("DisabledEnum"=w291) -> ()  [unwired: 2 in, 2 out]
    n334 = case shown="True" w176 {
      tunnel: [_ "i"] -> w482
      frame False {
      }
      frame True {
      }
    }
    n335 = case shown="True" w179 {
      tunnel: [_ "t"] -> w481
      frame False {
      }
      frame True {
      }
    }
    n336 = case shown="True" w433 {
      tunnel: [_ "a" ("write buffer")] -> w478
      frame False {
      }
      frame True {
        # "Send 'a' ABORT"
        n337 = property on="Secondary Safety" class="Bool (strict)"("Value"=TRUE) -> ()  [unwired: 2 in, 2 out]
      }
    }
    n338 = case shown="True" w435 {
      tunnel: [_ "k" ("write buffer")] -> w495
      frame False {
      }
      frame True {
        # "Send 'k' softkill"
      }
    }
    n339 = case shown="True" "Fan Shutdown" {
      tunnel: [_ "f"] -> w173
      frame False {
      }
      frame True {
        # "Sends 'f' to shut off fan"
      }
    }
    n340 = Array Size(array=w376) -> (size(s)=w375:i32)
    n341 = Index Array(array=w470, index=0) -> (element=w469:string)
    "String" <- w469
    n342 = Index Array(array=w376, index=0) -> (element=w519:string)
    n343 = Index Array(array=w376, index=7) -> (element=w508:string)
    n344 = Index Array(array=w376, index=1) -> (element=w518:string)
    n345 = Index Array(array=w376, index=8) -> (element=w507:string)
    n346 = Index Array(array=w376, index=2) -> (element=w517:string)
    n347 = Index Array(array=w376, index=9) -> (element=w506:string)
    n348 = Index Array(array=w376, index=3) -> (element=w516:string)
    n349 = Index Array(array=w376, index=4) -> (element=w515:string)
    n350 = Index Array(array=w376, index=5) -> (element=w514:string)
    n351 = Index Array(array=w376, index=6) -> (element=w476:string)
    n352 = Index Array(array=w376, index=13) -> (element=w499:string)
    n353 = Index Array(array=w376, index=10) -> (element=w504:string)
    n354 = Index Array(array=w376, index=11) -> (element=w503:string)
    n355 = Index Array(array=w376, index=12) -> (element=w502:string)
    n356 = Index Array(array=w376, index=16) -> (element=w418:string)
    n357 = Index Array(array=w376, index=14) -> (element=w420:string)
    n358 = Index Array(array=w376, index=15) -> (element=w419:string)
    n359 = Index Array(array=w376, index=17) -> (element=w417:string)
    n360 = Fract/Exp String To Number(string=w519) -> (number=w314:dbl)  [unwired: 3 in, 1 out]
    n361 = Fract/Exp String To Number(string=w518) -> (number=w313:dbl)  [unwired: 3 in, 1 out]
    n362 = Fract/Exp String To Number(string=w517) -> (number=w312:dbl)  [unwired: 3 in, 1 out]
    n363 = Fract/Exp String To Number(string=w516) -> (number=w311:dbl)  [unwired: 3 in, 1 out]
    n364 = Fract/Exp String To Number(string=w499) -> (number=w255:dbl)  [unwired: 3 in, 1 out]
    n365 = Fract/Exp String To Number(string=w515) -> (number=w310:dbl)  [unwired: 3 in, 1 out]
    n366 = Fract/Exp String To Number(string=w514) -> (number=w309:dbl)  [unwired: 3 in, 1 out]
    n367 = Fract/Exp String To Number(string=w476) -> (number=w308:dbl)  [unwired: 3 in, 1 out]
    n368 = Fract/Exp String To Number(string=w418) -> (number=w193:dbl)  [unwired: 3 in, 1 out]
    n369 = Fract/Exp String To Number(string=w420) -> (number=w207:dbl)  [unwired: 3 in, 1 out]
    n370 = Fract/Exp String To Number(string=w419) -> (number=w202:dbl)  [unwired: 3 in, 1 out]
    n371 = Fract/Exp String To Number(string=w417) -> (number=w188:dbl)  [unwired: 3 in, 1 out]
    n372 = Decrement(x=w375) -> (x-1=w374:i32)
    n373 = Fract/Exp String To Number(string=w508) -> (number=w254:dbl)  [unwired: 3 in, 1 out]
    "TCpw-1" <- w254
    n374 = Fract/Exp String To Number(string=w507) -> (number=w253:dbl)  [unwired: 3 in, 1 out]
    "TCpw-2" <- w253
    n375 = Fract/Exp String To Number(string=w506) -> (number=w252:dbl)  [unwired: 3 in, 1 out]
    "TCpw-3" <- w252
    n376 = Fract/Exp String To Number(string=w504) -> (number=w251:dbl)  [unwired: 3 in, 1 out]
    "TCpw-4" <- w251
    n377 = Fract/Exp String To Number(string=w503) -> (number=w248:dbl)  [unwired: 3 in, 1 out]
    "TCp-1" <- w248
    n378 = Fract/Exp String To Number(string=w502) -> (number=w247:dbl)  [unwired: 3 in, 1 out]
    "TCp-2" <- w247
    n379 = local read "Multiplier 1"() -> (w341:dbl)
    n380 = local read "Multiplier 2"() -> (w339:dbl)
    n381 = local read "Multiplier 3"() -> (w337:dbl)
    n382 = local read "Multiplier 4"() -> (w335:dbl)
    n383 = local read "Multiplier 5"() -> (w333:dbl)
    n384 = local read "Multiplier 6"() -> (w330:dbl)
    n385 = Equal?(x=w469, y="String 3") -> (x = y?=→"?":bool)
    n386 = Index Array(array=w376, index=w374) -> (element=w379:string)
    n387 = Concatenate Strings("h" ("string"), ":" ("string"), w498, w497, w496, w483, w494, w493, w492, w495, w482, w481, w480, w478, w479, w173, ";" ("string")) -> (w425:string)
    "Output" <- w425
    n388 = Divide(x=w207, y=10.0) -> (x/y=w205:dbl)
    n389 = Divide(x=w202, y=10.0) -> (x/y=w198:dbl)
    n390 = Divide(x=w193, y=10.0) -> (x/y=w195:dbl)
    n391 = Divide(x=w188, y=10.0) -> (x/y=w190:dbl)
    n392 = local read "Multiplier 7"() -> (w328:dbl)
    n393 = Subtract(x=w205, y=100.0) -> (x-y=→"Engine 1":dbl)
    n394 = Subtract(x=w195, y=100.0) -> (x-y=→"Engine 3":dbl)
    n395 = Subtract(x=w190, y=100.0) -> (x-y=→"Engine 4":dbl)
    n396 = Multiply(x=w314, y=w341) -> (x*y=w348:dbl)
    n397 = Multiply(x=w313, y=w339) -> (x*y=w347:dbl)
    n398 = Multiply(x=w312, y=w337) -> (x*y=w346:dbl)
    n399 = Multiply(x=w311, y=w335) -> (x*y=w345:dbl)
    n400 = Multiply(x=w310, y=w333) -> (x*y=w344:dbl)
    n401 = Multiply(x=w309, y=w330) -> (x*y=w343:dbl)
    n402 = Subtract(x=w198, y=100.0) -> (x-y=→"Engine 2":dbl)
    n403 = Bundle(w207, w202, w193, w188) -> (→"Motors":cluster{dbl, dbl, dbl, dbl})  [unwired: 1 in]
    n404 = Equal?(x=w254, y=-1.0) -> (x = y?=→"TC1":bool)
    n405 = Equal?(x=w254, y=-3.0) -> (x = y?=→"vcc":bool)
    n406 = Equal?(x=w254, y=-2.0) -> (x = y?=→"gnd":bool)
    n407 = Equal?(x=w253, y=-2.0) -> (x = y?=→"gnd 2":bool)
    n408 = Equal?(x=w253, y=-3.0) -> (x = y?=→"vcc 2":bool)
    n409 = Equal?(x=w253, y=-1.0) -> (x = y?=→"TC2":bool)
    n410 = Equal?(x=w252, y=-3.0) -> (x = y?=→"vcc 3":bool)
    n411 = Equal?(x=w252, y=-2.0) -> (x = y?=→"gnd 3":bool)
    n412 = Equal?(x=w252, y=-1.0) -> (x = y?=→"TC3":bool)
    n413 = Equal?(x=w251, y=-2.0) -> (x = y?=→"gnd 4":bool)
    n414 = Equal?(x=w251, y=-1.0) -> (x = y?=→"TC4":bool)
    n415 = Equal?(x=w251, y=-3.0) -> (x = y?=→"vcc 4":bool)
    n416 = Equal?(x=w248, y=-3.0) -> (x = y?=→"vcc 5":bool)
    n417 = Equal?(x=w248, y=-2.0) -> (x = y?=→"gnd 5":bool)
    n418 = Equal?(x=w248, y=-1.0) -> (x = y?=→"TC5":bool)
    n419 = Equal?(x=w247, y=-3.0) -> (x = y?=→"vcc 6":bool)
    n420 = Equal?(x=w247, y=-1.0) -> (x = y?=→"TC6":bool)
    n421 = Equal?(x=w247, y=-2.0) -> (x = y?=→"gnd 6":bool)
    n422 = Index Array(array=w376, index=18) -> (element=w318:string)
    n423 = Fract/Exp String To Number(string=w379) -> (number=→"ms":dbl)  [unwired: 3 in, 1 out]
    n424 = Equal?(x=w425, y=w318) -> (x = y?=w427:bool)
    n425 = Multiply(x=w308, y=w328) -> (x*y=w342:dbl)
    n426 = Search/Split String(string=w318, search string/char (-)="r") -> (offset of match=w365:i32)  [unwired: 1 in, 2 out]
    n427 = Search/Split String(string=w318, search string/char (-)="z") -> (offset of match=w367:i32)  [unwired: 1 in, 2 out]
    n428 = Search/Split String(string=w318, search string/char (-)="s") -> (offset of match=w369:i32)  [unwired: 1 in, 2 out]
    n429 = Search/Split String(string=w318, search string/char (-)="k") -> (offset of match=w431:i32)  [unwired: 1 in, 2 out]
    n430 = Search/Split String(string=w318, search string/char (-)="a") -> (offset of match=w372:i32)  [unwired: 1 in, 2 out]
    n431 = Search/Split String(string=w318, search string/char (-)="t") -> (offset of match=w361:i32)  [unwired: 1 in, 2 out]
    n432 = case shown="False" w427 {
      tunnel: [w592 _] -> w426
      tunnel: w425 -> [w592 _]
      frame False {
      }
      frame True {
      }
    }
    n433 = local read "Offset 1"() -> (w340:dbl)
    n434 = local read "Offset 2"() -> (w338:dbl)
    n435 = local read "Offset 3"() -> (w336:dbl)
    n436 = local read "Offset 4"() -> (w334:dbl)
    n437 = local read "Offset 5"() -> (w332:dbl)
    n438 = local read "Offset 6"() -> (w331:dbl)
    n439 = local read "Offset 7"() -> (w329:dbl)
    n440 = Greater Or Equal To 0?(x=w431) -> (x >= 0?=→"Craft Triggered Softkill Active":bool)
    n441 = Greater Or Equal To 0?(x=w372) -> (x >= 0?=w298:bool)
    "Hardkill Active" <- w298
    n442 = Greater Or Equal To 0?(x=w365) -> (x >= 0?=w303:bool)
    "Reset Triggered" <- w303
    n443 = Greater Or Equal To 0?(x=w367) -> (x >= 0?=w327:bool)
    "Flight Control On" <- w327
    n444 = Greater Or Equal To 0?(x=w361) -> (x >= 0?=w356:bool)
    n445 = Greater Or Equal To 0?(x=w369) -> (x >= 0?=w357:bool)
    "Primary Safety Active" <- w357
    n446 = Multiply(x=0.0069, y=w255) -> (x*y=w256:dbl)
    n447 = Bundle(w254, w253, w252, w251) -> (→"?":cluster{dbl, dbl, dbl, dbl})  [unwired: 1 in]
    n448 = Bundle(w248, w247) -> (→"?":cluster{dbl, dbl})  [unwired: 1 in]
    n449 = local read "Manual Abort Tested"() -> (w362:bool)
    n450 = local read "Reset Triggered 2"() -> (w363:bool)
    n451 = Add(x=w340, y=w348) -> (x+y=w240:dbl)
    "PT4-M" <- w240
    n452 = Add(x=w338, y=w347) -> (x+y=w243:dbl)
    "PT1-M" <- w243
    n453 = Add(x=w336, y=w346) -> (x+y=w241:dbl)
    "PT3-M" <- w241
    n454 = Add(x=w334, y=w345) -> (x+y=w245:dbl)
    "PT1-U" <- w245
    n455 = Add(x=w332, y=w344) -> (x+y=w242:dbl)
    "PT2-U" <- w242
    n456 = Add(x=w331, y=w343) -> (x+y=w322:dbl)
    "PT2-M" <- w322
    n457 = Add(x=w329, y=w342) -> (x+y=w239:dbl)
    "PT5-M" <- w239
    n458 = Add(x=11.144, y=w256) -> (x+y=w238:dbl)
    "Voltage Sensor" <- w238
    "?" <- w238
    n459 = Or(x=w362, y=w298) -> (x .or. y?=w359:bool)
    "Manual Abort Tested" <- w359
    n460 = Or(x=w363, y=w303) -> (x .or. y?=w358:bool)
    "Reset Triggered 2" <- w358
    n461 = local read "PT1-U"() -> (w285:dbl)
    n462 = Build Array(w314, w313, w312, w311, w310, w309, w308, w240, w243, w241, w245, w242, w322, w239, w254, w253, w252, w251, w248, w247, w238, w207, w202, w202, w188) -> (w321:dbl[])
    n463 = Bundle(w238, w254, w253, w252, w251, w248, w247, w240, w243, w241, w245, w242, w322, w239) -> (w305:T3)  [unwired: 1 out]
    n464 = Subtract(x=w285, y=5000) -> (x-y=w286:dbl)
    n465 = Bundle(w245, w242) -> (→"?":cluster{dbl, dbl})  [unwired: 1 in]
    n466 = Greater Than 0?(x=w286) -> (x > 0?=→"PT1-U > 5000 PSI":bool)
    n467 = Build Array(w359, w358, w327, w356, w357) -> (w355:bool[])
    n468 = Bundle(w243, w242, w241, w240, w239) -> (→"?":cluster{dbl, dbl, dbl, dbl, dbl})  [unwired: 1 in]
    n469 = case shown="True" "Send" {
      tunnel: w373 -> [_ w699]
      tunnel: w426 -> [_ w698]
      tunnel: w304 -> [_ w697]
      frame False {
      }
      frame True {
        n470 = case shown="Error" w699 {
          selector: w699 -> [w702 w706]
          tunnel: [w704 w705] -> _
          tunnel: [w703 w706] -> _
          tunnel: w698 -> [w701 _]
          tunnel: w697 -> [w700 w705]
          frame No Error {
            n471 = VISA Write(VISA resource name=w700, write buffer=w701, error in (no error)=w702) -> (VISA resource name out=w704:refnum<visa-resource-name>, error out=w703:errorcluster)  [unwired: 1 out]
          }
          frame Error {
          }
        }
      }
    }
    n472 = Array To Spreadsheet String(delimiter (Tab)="\t", array=w321, 3:"%d" ("format string")) -> (spreadsheet string=w302:string)
    n473 = Max & Min(x=w306, y=w305) -> (max(x,y)=w307:T3)  [unwired: 1 out]
    "Max Values" <- w307
    n474 = And Array Elements(Boolean array=w355) -> (logical AND=w351:bool)
    n475 = Search/Split String(string=w302, search string/char (-)="\r\n") -> (substring before match=w300:string)  [unwired: 1 in, 2 out]
    n476 = And(x=w354, y=w351) -> (x .and. y?=w353:bool)
    n477 = Concatenate Strings(w300, "\t" ("string"), w318, "\n" ("string")) -> (w316:string)
    n478 = Or(x=w354, y=w353) -> (x .or. y?=w352:bool)
    n479 = Write to Text File(file (use dialog)=w326, text=w316) -> (refnum out=w323:refnum<file>)  [unwired: 2 in, 2 out]
    n480 = Exclusive Or(1:w352, 2:"Begin Checklist") -> (0:w370:bool)
    n481 = case shown="True" w370 {
      frame False {
      }
      frame True {
        w591 = FALSE
        n482 = local write "Reset Triggered 2"(w591) -> ()
        n483 = local write "Manual Abort Tested"(w591) -> ()
      }
    }
    n484 = Wait Until Next ms Multiple(millisecond multiple=200) -> ()  [unwired: 1 out]
    "Iterations" <- w292
  }
  n485 = VISA Open(VISA resource name=refnum<visa-resource-name> "COM3") -> (VISA resource name=w5:refnum<visa-resource-name>, error out=w4:errorcluster)  [unwired: 4 in]
  n486 = VISA Close(VISA resource name=w5, error in (no error)=w4) -> ()  [unwired: 1 out]
  n487 = VISA Close(VISA resource name=w7, error in (no error)=w61) -> ()  [unwired: 1 out]
  n488 = Close File(refnum=w58) -> ()  [unwired: 1 in, 2 out]
